vi "labview parse dist.vi"(10 "Telegram String":string) -> (2 "Angle Array":dbl[](array[numeric]), 3 "Distance Array":u32[](array[numeric]))   [LabVIEW 2017]
panel:
  out "Reversed Angle Array":bool=TRUE
  out "Angular Step":dbl
  out "Angle Start":dbl
  out "Amount of data":u32
  out "Telegram Array":string[](array[string])
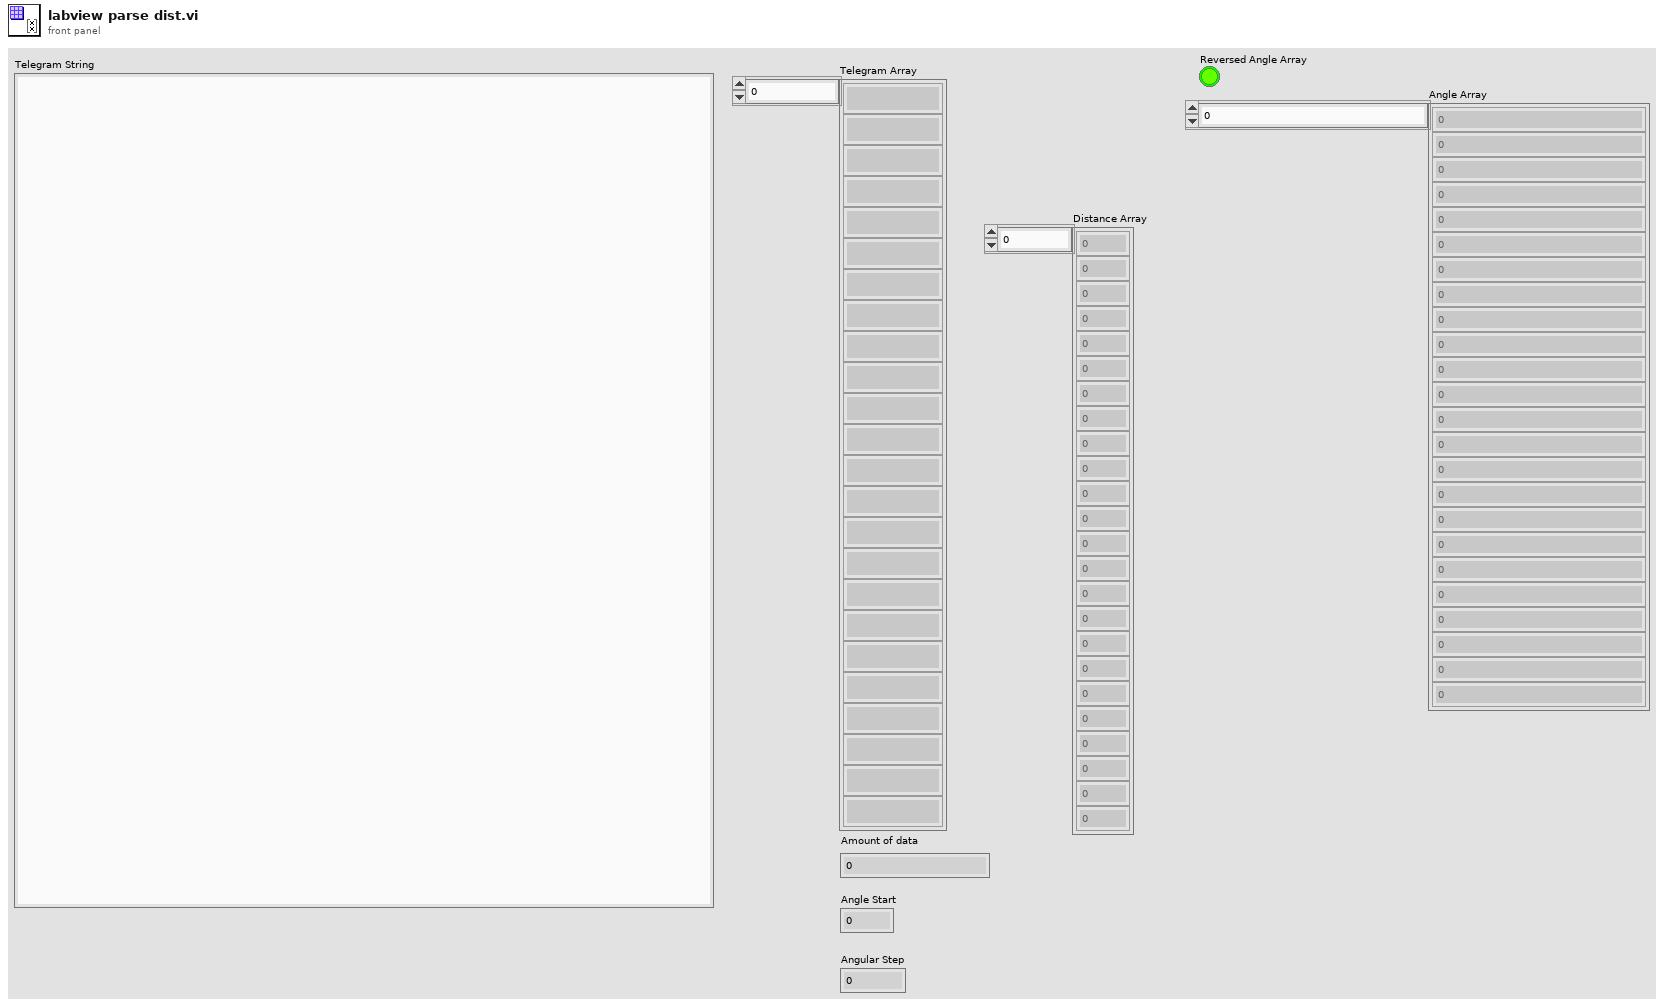
[diagram p1: front panel]
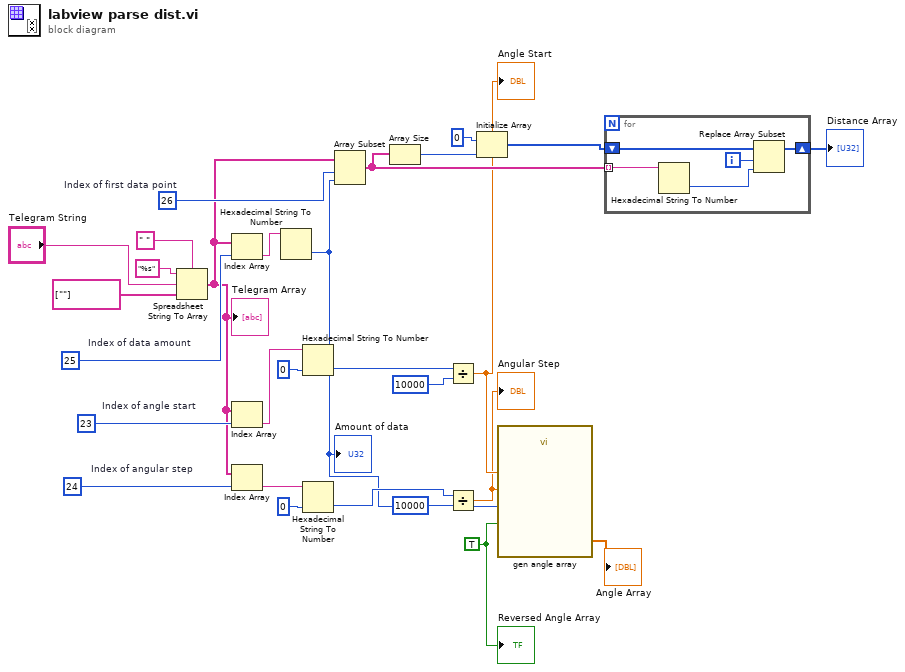
[diagram p0: block diagram]
diagram:
  w2 = TRUE
  w8 = 24  # Index of angular step
  w13 = 23  # Index of angle start
  w19 = 25  # Index of data amount
  w25 = 26  # Index of first data point
  n1 = Spreadsheet String To Array(delimiter (Tab)=" ", format string="%s", spreadsheet string="Telegram String", array type (2D Dbl)=string[] [""]) -> (array=w7:string[])
  "Telegram Array" <- w7
  n2 = Index Array(array=w7, index=w19) -> (element=w18:string)
  n3 = Index Array(array=w7, index=w13) -> (element=w14:string)
  n4 = Index Array(array=w7, index=w8) -> (element=w9:string)
  n5 = Hexadecimal String To Number(string=w18) -> (number=w4:u32)  [unwired: 2 in, 1 out]
  "Amount of data" <- w4
  n6 = Hexadecimal String To Number(string=w14, default (0uL)=0 ("default (0 U32)")) -> (number=w16:i32)  [unwired: 1 in, 1 out]
  n7 = Hexadecimal String To Number(string=w9, default (0uL)=0 ("default (0 U32)")) -> (number=w11:i32)  [unwired: 1 in, 1 out]
  n8 = Array Subset(array=w7, index=w25, length=w4) -> (w23:string[])
  n9 = Array Size(array=w23) -> (size(s)=w24:i32)
  n10 = Divide(x=w16, y=10000) -> (x/y=w6:dbl)
  "Angle Start" <- w6
  n11 = Divide(x=w11, y=10000) -> (x/y=w5:dbl)
  "Angular Step" <- w5
  n12 = Initialize Array(u32 0 ("element"), w24) -> (w21:u32[])
  n13 = call "gen angle array.vi"("Invert"=w2, "angular step"=w5, "angle start"=w6, "array size"=w4) -> ("output array"=→"Angle Array":dbl[])  [unwired: 7 in]
  n14 = for {
    tunnel: w23 -> [w33] mode=indexing
    shift-right: [w29] -> w20
    shift-left: w21 -> [w30]
    i -> [w32]
    n15 = Hexadecimal String To Number(string=w33) -> (number=w31:u32)  [unwired: 2 in, 1 out]
    n16 = Replace Array Subset(array=w30, new element=w31, index=w32) -> (w29:u32[])
  }
  "Distance Array" <- w20
  "Reversed Angle Array" <- w2
